vi "Parse String.vi"(7 "conversion blocks":T1[](array[typedef]) {"string block descriptor"."buffer offset" format="%d bytes"; "engine block descriptor"."buffer offset" format="%d bytes"}, 8 "error in (no error)":errorcluster, 10 "dst buffer in":string, 11 "src buffer in":string) -> (0 "error out":errorcluster, 2 "dst buffer out":string, 3 "src buffer out":string)   [LabVIEW 2017, in "String Type Buffer Converter.lvlib" / "String Type Buffer Converter.lvclass"]
uses:
  String Type Buffer Converter.lvclass
  Conversion Block.ctl
  Builds/Data Sharing Framework/Current/Data Sharing Framework Core/DSF Core.lvlibp/Engine/Classes/Buffer Converter/Channel Descriptor.ctl
  Builds/Data Sharing Framework/Current/Data Sharing Framework Core/DSF Core.lvlibp/DSF Configuration API/Public/Controls/DSF Data Type.ctl
  Builds/Data Sharing Framework/Current/Data Sharing Framework Core/DSF Core.lvlibp
  Builds/Data Sharing Framework/Current/Data Sharing Framework Core/DSF Core.lvlibp/Engine/Classes/Buffer/Buffer.lvclass
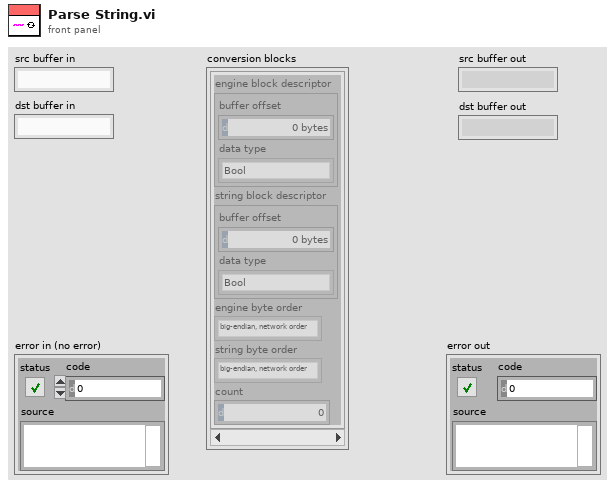
[diagram p1: front panel]
types:
  T1 = typedef "String Type Buffer Converter.lvlib/String Type Buffer Converter.lvclass/Conversion Block.ctl" = cluster{"engine block descriptor":T2, "string block descriptor":T2, "engine byte order":enum16{"big-endian, network order", "native, host order", "little-endian"}, "string byte order":enum16{"big-endian, network order", "native, host order", "little-endian"}, "count":u64}
  T2 = typedef "DSF Core.lvlibp/Buffer.lvclass/Channel Descriptor.ctl" = cluster{"buffer offset":u64, "data type":T3}
  T3 = typedef "DSF Core.lvlibp/DSF Data Type.ctl" = enum8{"Bool", "SGL", "DBL", "I8", "I16", "I32", "I64", "U8", "U16", "U32", "U64"}
  T4 = enum16{"big-endian, network order", "native, host order", "little-endian"}
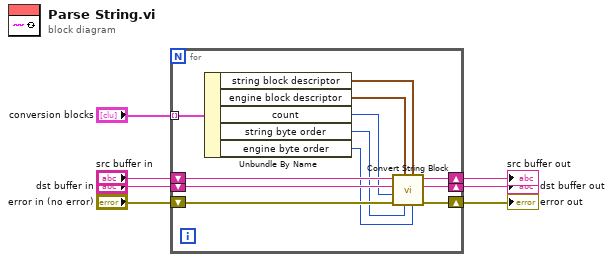
[diagram p0: block diagram]
diagram:
  n1 = for {
    tunnel: "conversion blocks" -> [w18] mode=indexing
    shift-right: [w15] -> w3
    shift-left: "error in (no error)" -> [w19]
    shift-right: [w14] -> w7
    shift-left: "dst buffer in" -> [w12]
    shift-right: [w13] -> w6
    shift-left: "src buffer in" -> [w11]
    n2 = Unbundle By Name(w18) -> ("string block descriptor"=w17:T2, "engine block descriptor"=w16:T2, "count"=w8:u64, "string byte order"=w9:T4, "engine byte order"=w10:T4)
    n3 = call "Convert String Block.vi"("dst byte order"=w10, "src block descriptor"=w17, "src byte order"=w9, "dst block descriptor"=w16, "error in (no error)"=w19, "channel count"=w8, "dst buffer in"=w12, "src buffer in"=w11) -> ("error out"=w15:errorcluster, "dst buffer out"=w14:string, "src buffer out"=w13:string)  [unwired: 1 in]
  }
  "src buffer out" <- w6
  "dst buffer out" <- w7
  "error out" <- w3
